vi "Get Coord Translation Vector.vi"(11 "Obstacle Avoidance Data":T1) -> (3 "Translation Vector":cluster{"X":dbl, "Y":dbl})   [LabVIEW 2017]
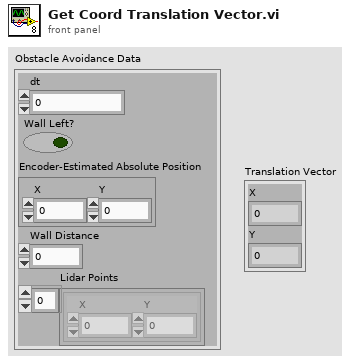
[diagram p1: front panel]
types:
  T1 = cluster{"dt":dbl, "Wall Left?":bool, "Encoder-Estimated Absolute Position":cluster{"X":dbl, "Y":dbl}, "Wall Distance":dbl, "Lidar Points":cluster{"X":dbl, "Y":dbl}[]}
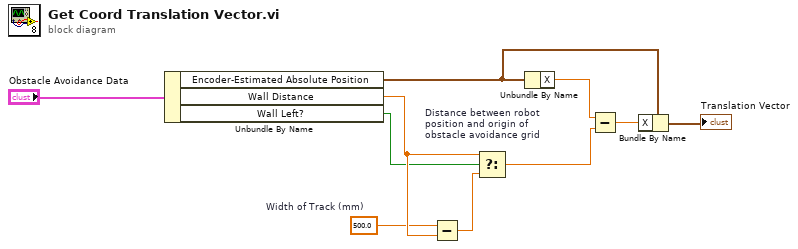
[diagram p0: block diagram]
diagram:
  w3 = 500.0  # Width of Track (mm)
  n1 = Unbundle By Name("Obstacle Avoidance Data") -> ("Encoder-Estimated Absolute Position"=w10:cluster{"X":dbl, "Y":dbl}, "Wall Distance"=w4:dbl, "Wall Left?"=w2:bool)
  n2 = Subtract(x=w3, y=w4) -> (x-y=w5:dbl)
  n3 = Select "Distance between robot position and origin of obstacle avoidance grid"(t=w4, s=w2, f=w5) -> (s? t:f=w6:dbl)
  n4 = Unbundle By Name(w10) -> ("X"=w7:dbl)
  n5 = Subtract(x=w7, y=w6) -> (x-y=w8:dbl)
  n6 = Bundle By Name(cluster=w10, "X"=w8) -> (→"Translation Vector":cluster{"X":dbl, "Y":dbl})
